vi "MMtoDD.vi"(9 "输入的四位小数毫米值":dbl) -> (0 "双D输出":string[](array[string]), 1 "D值字符串":string)   [LabVIEW 2015]
panel:
  out "十六进制整型字符串":string
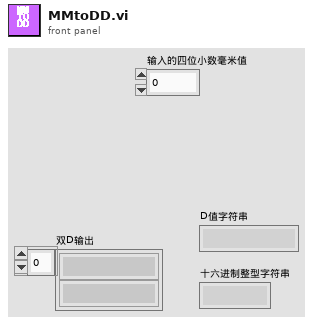
[diagram p1: front panel]
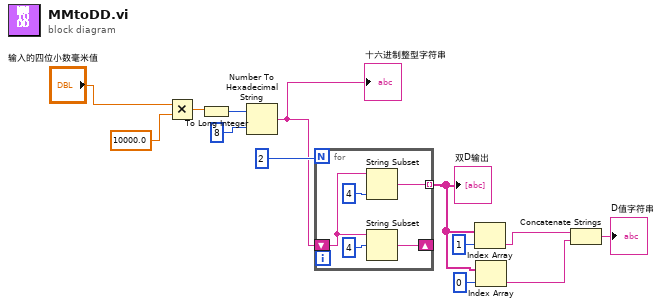
[diagram p0: block diagram]
diagram:
  n1 = Multiply(x="输入的四位小数毫米值", y=10000.0) -> (x*y=w11:dbl)
  n2 = To Long Integer(number=w11) -> (32bit integer=w10:i32)
  n3 = Number To Hexadecimal String ("数值至十六进制字符串转换")(1:i16 8 ("宽度(-)"), 2:w10) -> (0:w8:string)
  "十六进制整型字符串" <- w8
  n4 = for {
    N: 2 -> [_]
    tunnel: [w15] -> w5 mode=indexing
    shift-right: [w17] -> _
    shift-left: w8 -> [w14]
    n5 = String Subset(string=w14, length (rest)=4 ("长度（剩余）")) -> (substring=w15:string)  [unwired: 1 in]
    n6 = String Subset(string=w14, offset (0)=4 ("长度（剩余）")) -> (substring=w17:string)  [unwired: 1 in]
  }
  "双D输出" <- w5
  n7 = Index Array(array=w5, index=1 ("索引")) -> (element=w4:string)
  n8 = Index Array(array=w5, index=0 ("索引")) -> (element=w3:string)
  n9 = Concatenate Strings(w4, w3) -> (→"D值字符串":string)
